vi "2-html-账户信息-数组btc - 副本.vi"(11 "body":string caption="体部") -> (3 "账户信息":string[](array[string]))   [LabVIEW 2020]
panel:
  out "receive":string
  out "last":string
  out "balanceusd":string
  out "balance":string
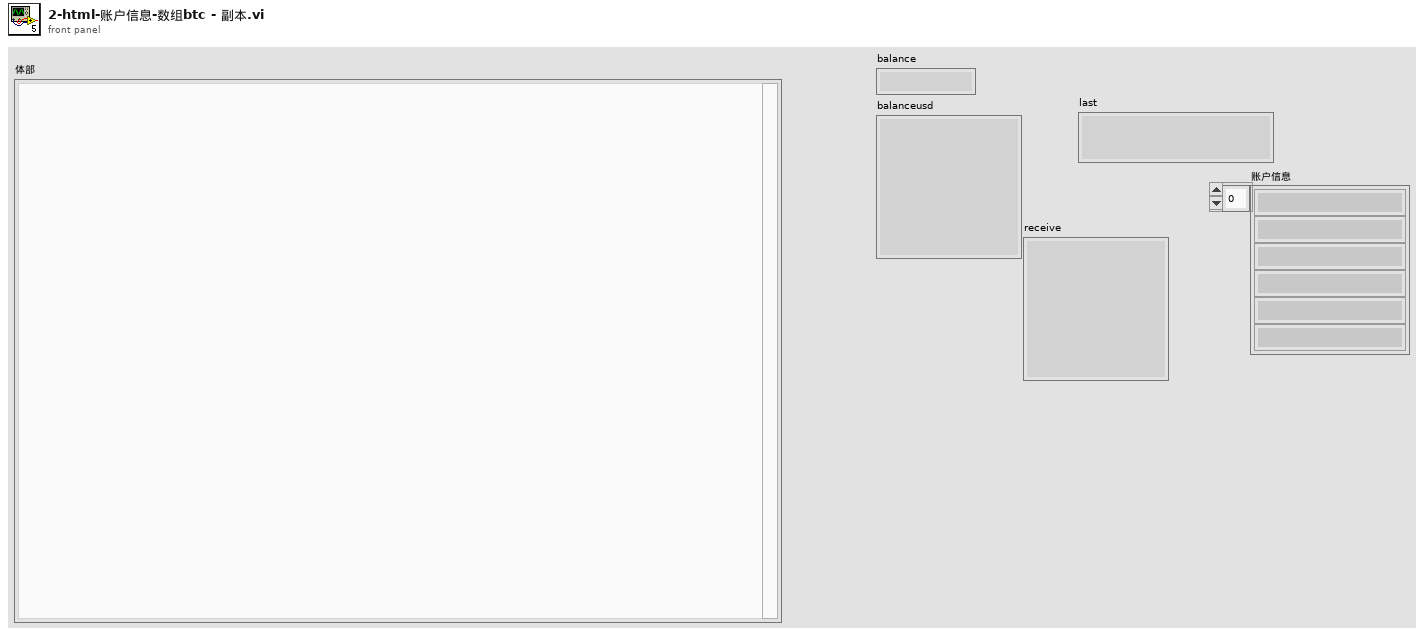
[diagram p1: front panel]
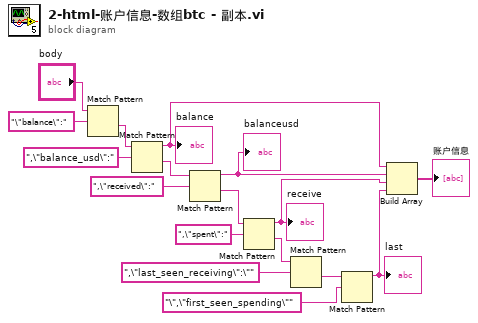
[diagram p0: block diagram]
diagram:
  n1 = Match Pattern(string="body", regular expression="\"balance\":") -> (after substring=w15:string)  [unwired: 1 in, 3 out]
  n2 = Match Pattern(string=w15, regular expression=",\"balance_usd\":" ("正则表达式")) -> (before substring=w8:string, after substring=w10:string)  [unwired: 1 in, 2 out]
  "balance" <- w8
  n3 = Match Pattern(string=w10, regular expression=",\"received\":" ("正则表达式")) -> (before substring=w3:string, after substring=w6:string)  [unwired: 1 in, 2 out]
  "balanceusd" <- w3
  n4 = Match Pattern(string=w6, regular expression=",\"spent\":" ("正则表达式")) -> (before substring=w2:string, after substring=w4:string)  [unwired: 1 in, 2 out]
  "receive" <- w2
  n5 = Match Pattern(string=w4, regular expression=",\"last_seen_receiving\":\"" ("正则表达式")) -> (after substring=w12:string)  [unwired: 1 in, 3 out]
  n6 = Match Pattern(string=w12, regular expression="\",\"first_seen_spending\"" ("正则表达式")) -> (before substring=w1:string)  [unwired: 1 in, 3 out]
  "last" <- w1
  n7 = Build Array(w8, w3, w2, w1) -> (→"账户信息":string[])
